vi "M08 T.V.vi"(11 "NXT/EV3":T1) -> (3 "EV3 out":T1)   [LabVIEW 2016]
uses:
  <vilib>/NXT/Subs/LVHSConnector.ctl
  <vilib>/NXT/LegoClasses/BrickReference/BrickReference.lvclass
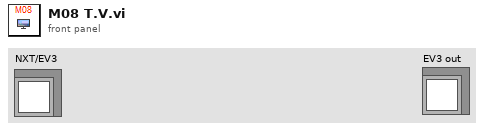
[diagram p1: front panel]
types:
  T1 = typedef "LVHSConnector.ctl" = refnum<class "BrickReference.lvclass">
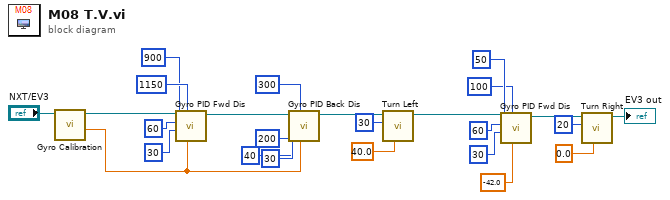
[diagram p0: block diagram]
diagram:
  n1 = call "Gyro Calibration.vi"("NXT/EV3"="NXT/EV3") -> ("Degrees"=w17:sgl, "NXT/EV3"=w25:T1)  [unwired: 6 in, 1 out]
  n2 = call "Gyro PID Fwd Dis.vi"("Target angle"=w17, "Threshold to stop"=1150, "Threshold to slow"=900, "Min. speed"=30, "Max. speed"=60, "EV3 in"=w25) -> ("EV3 out"=w20:T1)  [unwired: 5 in]
  n3 = call "Gyro PID Back Dis.vi"("Target angle"=w17, "Threshold to stop"=300, "Threshold to slow"=200, "Min. speed"=30, "Max. speed"=40, "EV3 in"=w20) -> ("EV3 out"=w14:T1)  [unwired: 5 in]
  n4 = call "Turn Left.vi"("Turning angle"=sgl 40.0, "Motor B (right)"=i8 30, "EV3 in"=w14) -> ("EV3 out"=w7:T1)  [unwired: 8 in]
  n5 = call "Gyro PID Fwd Dis.vi"("Target angle"=sgl -42.0, "Threshold to stop"=100, "Threshold to slow"=50, "Min. speed"=30, "Max. speed"=60, "EV3 in"=w7) -> ("EV3 out"=w5:T1)  [unwired: 5 in]
  n6 = call "Turn Right.vi"("Turning angle"=sgl 0.0, "Motor B (right)"=i8 20, "EV3 in"=w5) -> ("EV3 out"=→"EV3 out":T1)  [unwired: 8 in]
